vi "HW_7p1_Task1_PRADHASK.vi"() -> ()   [LabVIEW 2016]
uses:
  <vilib>/express/express arith-compare/Formula/XNode/ExpressFormulaBlockNode.xnode
panel:
  out "Time period":dbl
  out "Updated n":dbl
  in  "Carrying Capacity K":dbl
  in  "Death Rate":dbl
  in  "Birth Rate":dbl
  in  "Initial Population n":dbl
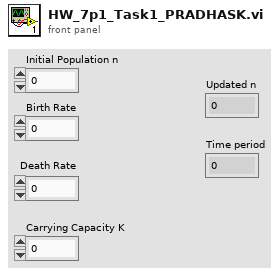
[diagram p1: front panel]
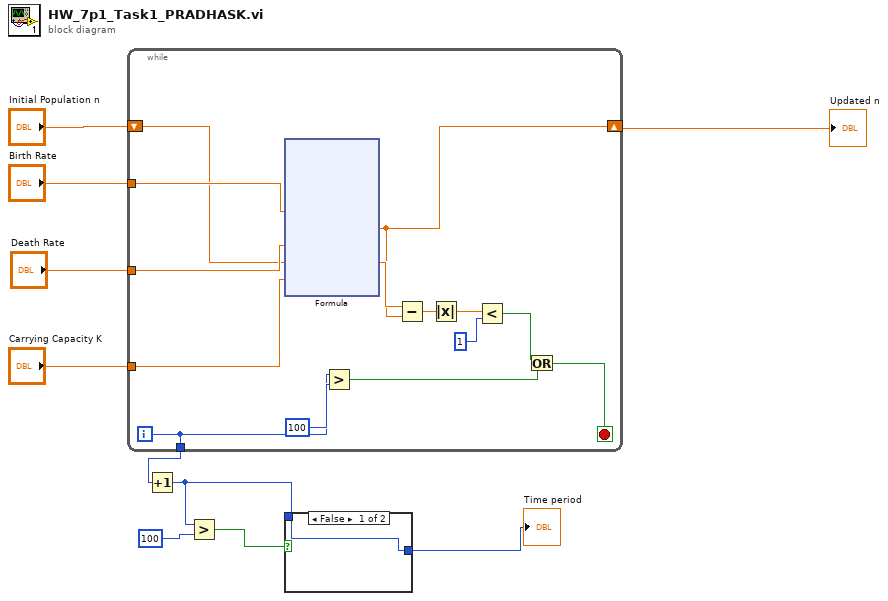
[diagram p0: block diagram]
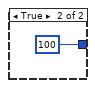
[diagram p2: hidden frame]
diagram:
  n1 = while {
    tunnel: "Birth Rate" -> [w23]
    tunnel: "Death Rate" -> [w22]
    tunnel: "Carrying Capacity K" -> [w21]
    shift-right: [w16] -> w6
    shift-left: "Initial Population n" -> [w20]
    tunnel: [w11] -> w3
    i -> [w11]
    stop <- w12 stop-if-true
    n2 = xnode "Formula"("BR"=w23, "DR"=w22, "n"=w20, "k"=w21) -> ("Result"=w16:dbl)  [unwired: 1 in, 1 out]
    n3 = Greater?(x=w11, y=100) -> (0:w13:bool)
    n4 = Subtract(x=w20, y=w16) -> (x-y=w17:dbl)
    n5 = Absolute Value(x=w17) -> (abs(x)=w19:dbl)
    n6 = Less?(x=w19, y=1) -> (x < y?=w14:bool)
    n7 = Or(x=w14, y=w13) -> (x .or. y?=w12:bool)
  }
  "Updated n" <- w6
  n8 = Increment(x=w3) -> (x+1=w1:i32)
  n9 = Greater?(x=w1, y=100) -> (0:w4:bool)
  n10 = case shown="False" w4 {
    tunnel: [w38 100] -> w2
    tunnel: w1 -> [w38 _]
    frame False {
    }
    frame True {
    }
  }
  "Time period" <- w2
